vi "DL-SMART-MS-Modify-03-16.vi"() -> ()   [LabVIEW 2013]
uses:
  resources.vi
panel:
  out "status":string
  out "source":string
  out "DI":bool[](array[boolean])
  out "AI":dbl[](array[numeric])
  in  "message":string
  in  "offset Y":dbl format="%#_13g"
  in  "offset X":dbl format="%#_13g"
  out "ADC aquiring":bool
  out "motor moving":bool
  out "busy":bool
  out "Pul.HV-Real":dbl
  in  "ReportResult":bool
  out "Identify Spcetrum":cluster{"all rows":dbl[], "all rows":dbl[]}[](graph)=[{"all rows"=array[50131 elements], "all rows"=array[50131 elements]}, {"all rows"=array[360 elements], "all rows"=[0.0, -15.85746, 0.0, 0.0, -4.11823, 0.0, 0.0, -20.55303, 0.0, 0.0, -3.65583, 0.0, 0.0, -2.69345, 0.0, 0.0, -4.4706, 0.0, 0.0, -6.07537, 0.0, 0.0, -4.25015, 0.0, 0.0, -6.95758, 0.0, 0.0, -2.04252, 0.0, 0.0, -7.70754, 0.0, 0.0, -4.28864, 0.0, 0.0, -4.00869, 0.0, 0.0, -4.47517, 0.0, 0.0, -14.21368, 0.0, 0.0, -6.66072, 0.0, 0.0, -6.50078, 0.0, 0.0, -3.75903, 0.0, 0.0, -17.29715, 0.0, 0.0, -6.92254, 0.0, 0.0, -2.52353, 0.0, 0.0, -3.06405, 0.0, 0.0, -16.54211, 0.0, 0.0, -5.10076, 0.0, 0.0, -8.01669, 0.0, 0.0, -40.71695, 0.0, 0.0, -4.03763, 0.0, 0.0, -3.14159, 0.0, 0.0, -2.79298, 0.0, 0.0, -13.41979, 0.0, 0.0, -7.6464, 0.0, 0.0, -6.18956, 0.0, 0.0, -2.44901, 0.0, 0.0, -5.1704, 0.0, 0.0, -3.62455, 0.0, 0.0, -6.443, 0.0, 0.0, -24.18432, 0.0, 0.0, -37.78631, 0.0, 0.0, -4.28528, 0.0, 0.0, -3.21654, 0.0, 0.0, -3.13522, 0.0, 0.0, -4.8477, 0.0, 0.0, -3.80614, 0.0, 0.0, -8.10386, 0.0, 0.0, -2.86382, 0.0, 0.0, -17.8978, 0.0, 0.0, -4.74503, 0.0, 0.0, -9.4855, 0.0, 0.0, -5.75364, 0.0, 0.0, -80.29859, 0.0, 0.0, -5.18928, 0.0, 0.0, -28.13783, 0.0, 0.0, -6.84449, 0.0, 0.0, -4.07742, 0.0, 0.0, -2.99391, 0.0, 0.0, -4.60838, 0.0, 0.0, -3.257, 0.0, 0.0, -5.79015, 0.0, 0.0, -24.98325, 0.0, 0.0, -4.30828, 0.0, 0.0, -5.54625, 0.0, 0.0, -5.47663, 0.0, 0.0, -100.0001, 0.0, 0.0, -21.11295, 0.0, 0.0, -12.03347, 0.0, 0.0, -6.35092, 0.0, 0.0, -4.71483, 0.0, 0.0, -6.58836, 0.0, 0.0, -3.41548, 0.0, 0.0, -3.10072, 0.0, 0.0, -4.79955, 0.0, 0.0, -4.88109, 0.0, 0.0, -32.02295, 0.0, 0.0, -20.17071, 0.0, 0.0, -9.63953, 0.0, 0.0, -8.63946, 0.0, 0.0, -6.018, 0.0, 0.0, -6.3389, 0.0, 0.0, -14.67808, 0.0, 0.0, -6.22948, 0.0, 0.0, -4.9166, 0.0, 0.0, -44.64096, 0.0, 0.0, -5.6163, 0.0, 0.0, -8.56872, 0.0, 0.0, -11.1186, 0.0, 0.0, -4.42493, 0.0, 0.0, -15.45284, 0.0, 0.0, -2.99091, 0.0, 0.0, -18.05376, 0.0, 0.0, -3.06669, 0.0, 0.0, -35.88844, 0.0, 0.0, -19.12645, 0.0, 0.0, -3.20878, 0.0, 0.0, -2.61247, 0.0, 0.0, -7.79975, 0.0, 0.0, -5.8874, 0.0, 0.0, -5.7487, 0.0, 0.0, -5.43834, 0.0, 0.0, -21.69908, 0.0, 0.0, -64.96584, 0.0, 0.0, -5.77762, 0.0, 0.0, -5.55465, 0.0, 0.0, -4.62119, 0.0, 0.0, -3.61176, 0.0, 0.0, -6.99332, 0.0, 0.0, -4.34549, 0.0, 0.0, -15.09003, 0.0, 0.0, -6.25437, 0.0, 0.0, -21.85243, 0.0, 0.0, -13.24381, 0.0, 0.0, -3.94672, 0.0, 0.0, -3.90192, 0.0, 0.0, -11.14967, 0.0, 0.0, -83.69183, 0.0, 0.0, -11.19559, 0.0, 0.0, -7.83445, 0.0, 0.0, -3.14763, 0.0, 0.0, -6.44728, 0.0, 0.0, -5.69155, 0.0, 0.0, -4.00216, 0.0]}]
  in  "IdentifyMS":bool
  out "Spcetrum":cluster{"all rows":dbl[], "all rows":dbl[]}(graph)
  in  "Identification Record (鉴定记录表)":i32(listbox)=6
  in  "Identification Results (单靶鉴定结果)":i32(listbox)=2
  out "RedLaserEnergy":sgl=3.5 format="%.1f"
  in  "HVEnable":bool
  in  "CameraSet":bool
  out "执行进度栏":u8(slide) caption="Vaccum" scale=0.0..1.0
  out "GateClose":bool
  out "LaserOK":bool
  out "HV-OK":bool
  out "Vacuum-OK":bool
  in  "Tab Control":T1(tab)
  in  "SumShots (累加总数)":u32=300
  in  "Evalu. Shots (评估数)":u32=100
  in  "螺线半径步长":dbl=1.0
  in  "螺线旋转角度":u32=30
  in  "EditAutoTar":bool
  in  "SinglePoint":bool=TRUE
  in  "MultiPoints":bool
  in  "MultiTargets":bool
  in  "MCPHV-Set":dbl
  in  "LensHV-Set":dbl
  in  "Tar.HV-Set":dbl
  in  "Pul.HV-Set":dbl
  in  "PulseDelay":dbl
  in  "ADCFreq":dbl
  in  "MassRange":cluster{u64, u64}(slide) scale=0.0..100000.0
  in  "CH1_Coupling":u64(ring)=2 items=["Volt DC"=1, "Volt AC"=2, "Ampere DC"=4, "Ampere AC"=8, "Ohm"=16]
  in  "Channel 1_Range":dbl(ring)=4.0 items=["80 V"=80.0, "40 V"=40.0, "20 V"=20.0, "8 V"=8.0, "4 V"=4.0, "2 V"=2.0, "800 mV"=0.8, "400 mV"=0.4, "200 mV"=0.2]
  in  "Anal. Setting File":string="High Mass"
  in  "SettingFileSave":bool caption="TakeMS"
  in  "SettingFileAppl":bool caption="TakeMS"
  in  "SettingDel":bool caption="TakeMS"
  in  "RunADC":bool caption="TakeMS"
  in  "StopADC":bool caption="TakeMS"
  out "ADCstatus":bool
  out "TurboPower":dbl[unit]
  out "TurboVolts":dbl[unit]
  out "TurboCurr":dbl[unit]
  out "TurboAge":dbl[unit]
  out "TurboTemp":dbl[unit]
  in  "TurboRun":bool caption="TakeMS"
  in  "TurboStop":bool caption="TakeMS"
  out "TurboStatus":bool
  out "TurboSpeed":dbl(knob) scale=0.0..100.0
  in  "Vac_Prot.":bool
  in  "Turbo_Fore":bool
  in  "Main_Samp":bool
  in  "Samp_Atmos":bool
  in  "Fore_Samp":bool
  in  "激光运行":bool caption="TakeMS"
  out "发射":bool
  in  "频率/Hz":u8=60
  in  "激光衰减偏置当前":u8
  in  "激光衰减偏置 2":u8
  in  "激光衰减偏置":u8
  out "欠压":bool
  out "过热":bool
  out "待机":bool
  out "连接":bool
  out "LaserVolt":sgl format="%.1f"
  out "LaserTemp":sgl format="%.1f"
  out "Numeric":i64
  out "温警":bool
  out "开关损坏":bool
  out "开关监控":bool
  out "命令":bool
  in  "激光停止":bool caption="TakeMS"
  in  "GO":bool
  out "YH12下":dbl
  out "YA1上":dbl
  out "XH12右":dbl
  out "XA1左":dbl
  in  "Y+":bool
  in  "Y-":bool
  in  "X-":bool
  in  "X+":bool
  in  "Plat_To_Zero":bool caption="TakeMS"
  in  "Plat_Cal":bool caption="TakeMS"
  out "Ty":dbl
  out "Tx":dbl
  out "Y当前":dbl
  out "X当前":dbl
  out "移动":bool
  out "Y满":bool
  out "Y标":bool
  out "X标":bool
  out "Y0":bool
  out "X0":bool
  out "靶位In/Out":bool
  out "仓门":bool
  out "Y过热":bool
  out "X过热":bool
  out "通讯":bool
  in  "Operation Record":i32(listbox)
  in  "OptionRecordLoad 2":bool caption="TakeMS"
  in  "OptionRecordClear":bool caption="TakeMS"
  in  "CameraStart":bool
  in  "OpenCloseGate":bool
  out "Camera (摄像头)":dbl[][](graph)
  out "Tar.HV-Real":dbl
  out "LensHV-Real":dbl
  out "MCPHV-Real":dbl
  out "Lvaccum":dbl=0.83 format="%#_6e"
  out "Hvaccum":dbl=3.4e-05 format="%#_6e"
  in  "H12":bool
  in  "G12":bool
  in  "F12":bool
  in  "E12":bool
  in  "D12":bool
  in  "C12":bool
  in  "B12":bool
  in  "A12":bool
  in  "H11":bool
  in  "G11":bool
  in  "F11":bool
  in  "E11":bool
  in  "D11":bool
  in  "C11":bool
  in  "B11":bool
  in  "A11":bool
  in  "H10":bool
  in  "G10":bool
  in  "F10":bool
  in  "E10":bool
  in  "D10":bool
  in  "C10":bool
  in  "B10":bool
  in  "A10":bool
  in  "H9":bool
  in  "G9":bool
  in  "F9":bool
  in  "E9":bool
  in  "D9":bool
  in  "C9":bool
  in  "B9":bool
  in  "A9":bool
  in  "H8":bool
  in  "G8":bool
  in  "F8":bool
  in  "E8":bool
  in  "D8":bool
  in  "C8":bool
  in  "B8":bool
  in  "A8":bool
  in  "H7":bool
  in  "G7":bool
  in  "F7":bool
  in  "E7":bool
  in  "D7":bool
  in  "C7":bool
  in  "B7":bool
  in  "A7":bool
  in  "H6":bool
  in  "G6":bool
  in  "F6":bool
  in  "E6":bool
  in  "D6":bool
  in  "C6":bool
  in  "B6":bool
  in  "A6":bool
  in  "H5":bool
  in  "G5":bool
  in  "F5":bool
  in  "E5":bool
  in  "D5":bool
  in  "C5":bool
  in  "B5":bool
  in  "A5":bool
  in  "H4":bool
  in  "G4":bool
  in  "F4":bool
  in  "E4":bool
  in  "D4":bool
  in  "C4":bool
  in  "B4":bool
  in  "A4":bool
  in  "H3":bool
  in  "G3":bool
  in  "F3":bool
  in  "E3":bool
  in  "D3":bool
  in  "C3":bool
  in  "B3":bool
  in  "A3":bool
  in  "H2":bool
  in  "G2":bool
  in  "F2":bool
  in  "E2":bool
  in  "D2":bool
  in  "C2":bool
  in  "B2":bool
  in  "A2":bool
  in  "H1":bool
  in  "G1":bool
  in  "F1":bool
  in  "E1":bool
  in  "D1":bool
  in  "C1":bool
  in  "B1":bool
  in  "A1":bool
  out "Added":u32=300
  out "ith-Shot":dbl
  in  "Clear":bool caption="TakeMS"
  in  "Add":bool caption="TakeMS"
  in  "TakeMS-Stop":bool caption="TakeMS"
  in  "TakeMS-Run":bool caption="TakeMS"
  out "Sumshots":u32=300
  in  "SetLaserEnergy":dbl(slide) scale=0.0..10.0
  # "Laser (激光)"
  # "Camera (摄像头)"
  # "Mass Spectrum (质谱图)"
  # "Energy"
  # "mJ/pulse"
  # "Acq.(采谱)"
  # "1"
  # "2"
  # "3"
  # "4"
  # "5"
  # "6"
  # "7"
  # "8"
  # "9"
  # "10"
  # "11"
  # "12"
  # "Vacuum(真空)"
  # "A"
  # "Pa"
  # "High"
  # "B"
  # "Low"
  # "Pa"
  # "C"
  # "H.V.(高压)"
  # "D"
  # "Ident. (鉴定图)"
  # "MCP"
  # "V"
  # "E"
  # "Tar."
  # "V"
  # "F"
  # "Pul."
  # "V"
  # "G"
  # "Lens"
  # "V"
  # "H"
  # "Vauum (真空)"
  # "H.V. (高压)"
  # "Laser (激光)"
  # "Gate (仓门)"
  # "SinglePoint (单点)"
  # "MultiPoints (多点)"
  # "MultiTar. (多靶)"
  # "mm"
  # "度"
  # "H.V. (高压参数)"
  # "ADC(采集卡设置)"
  # "ADCFreq(采样)"
  # "MCP (探测器)"
  # "V"
  # "Hz"
  # "Tar. (靶)"
  # "V"
  # "Setting File(设置文件)"
  # "Coupling"
  # "Pulse (脉冲)"
  # "V"
  # "IntRange"
  # "V"
  # "Lens (透镜)"
  # "Delay (延时)"
  # "ns"
  # "Turbo Pump"
  # "Sole. Valves"
  # "自锁保护"
  # "机械/分子"
  # "℃"
  # "主仓/样仓"
  # "样仓/大气"
  # "机械/样仓"
  # "激光器状态"
  # "激光衰减器："
  # "发射次数："
  # "偏置："
  # "温度："
  # "摄氏度"
  # "范围："
  # "内部电源电压："
  # "V"
  # "当前："
  # "um"
  # "um"
  # "um"
  # "um"
  # "um"
  # "um"
  # "度"
  # "度"
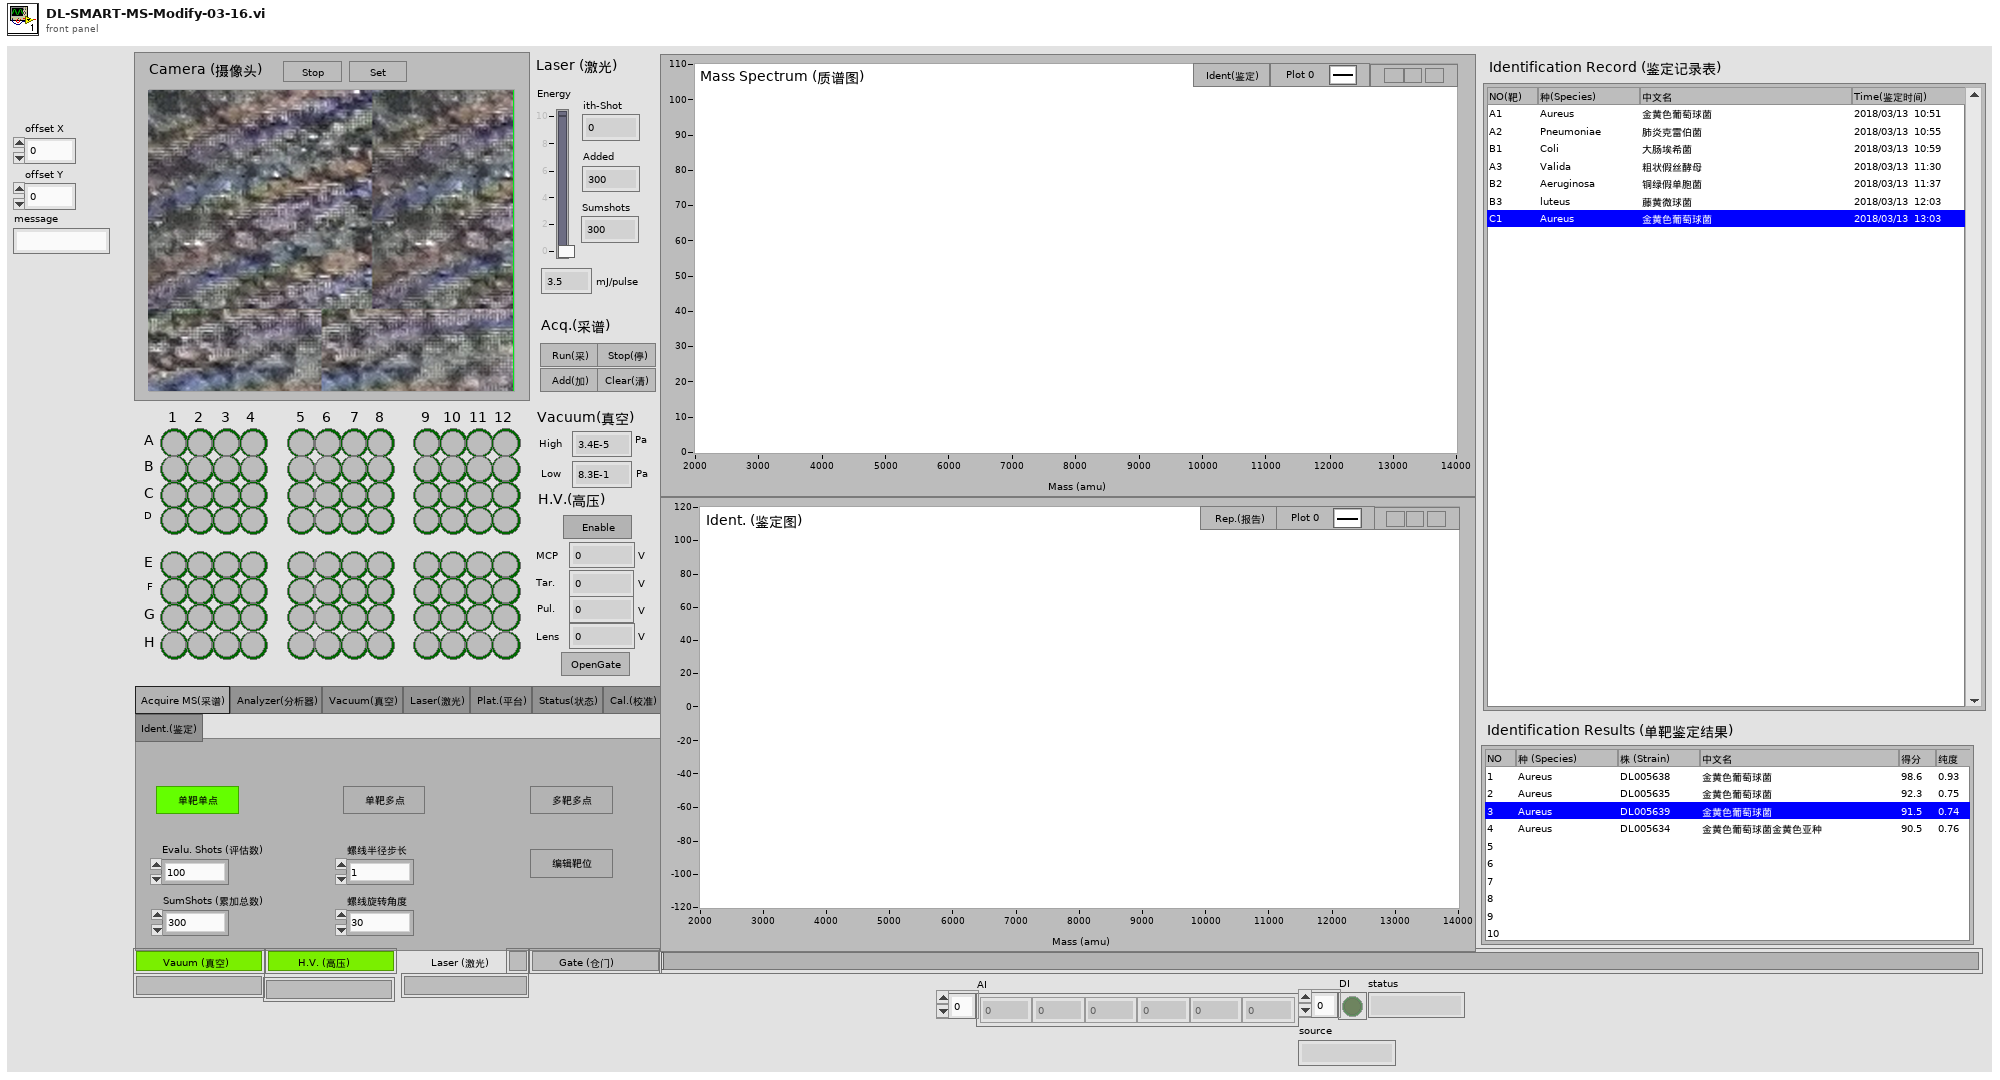
[diagram p1: front panel]
types:
  T1 = enum32{"Acquire MS(采谱)", "Analyzer(分析器)", "Vacuum(真空)", "Laser(激光)", "Plat.(平台)", "Status(状态)", "Cal.(校准)", "Ident.(鉴定)"}
  T2 = enum16{"adc aquire", "laser set", "motor move", "monitor", "wait", "stop"}
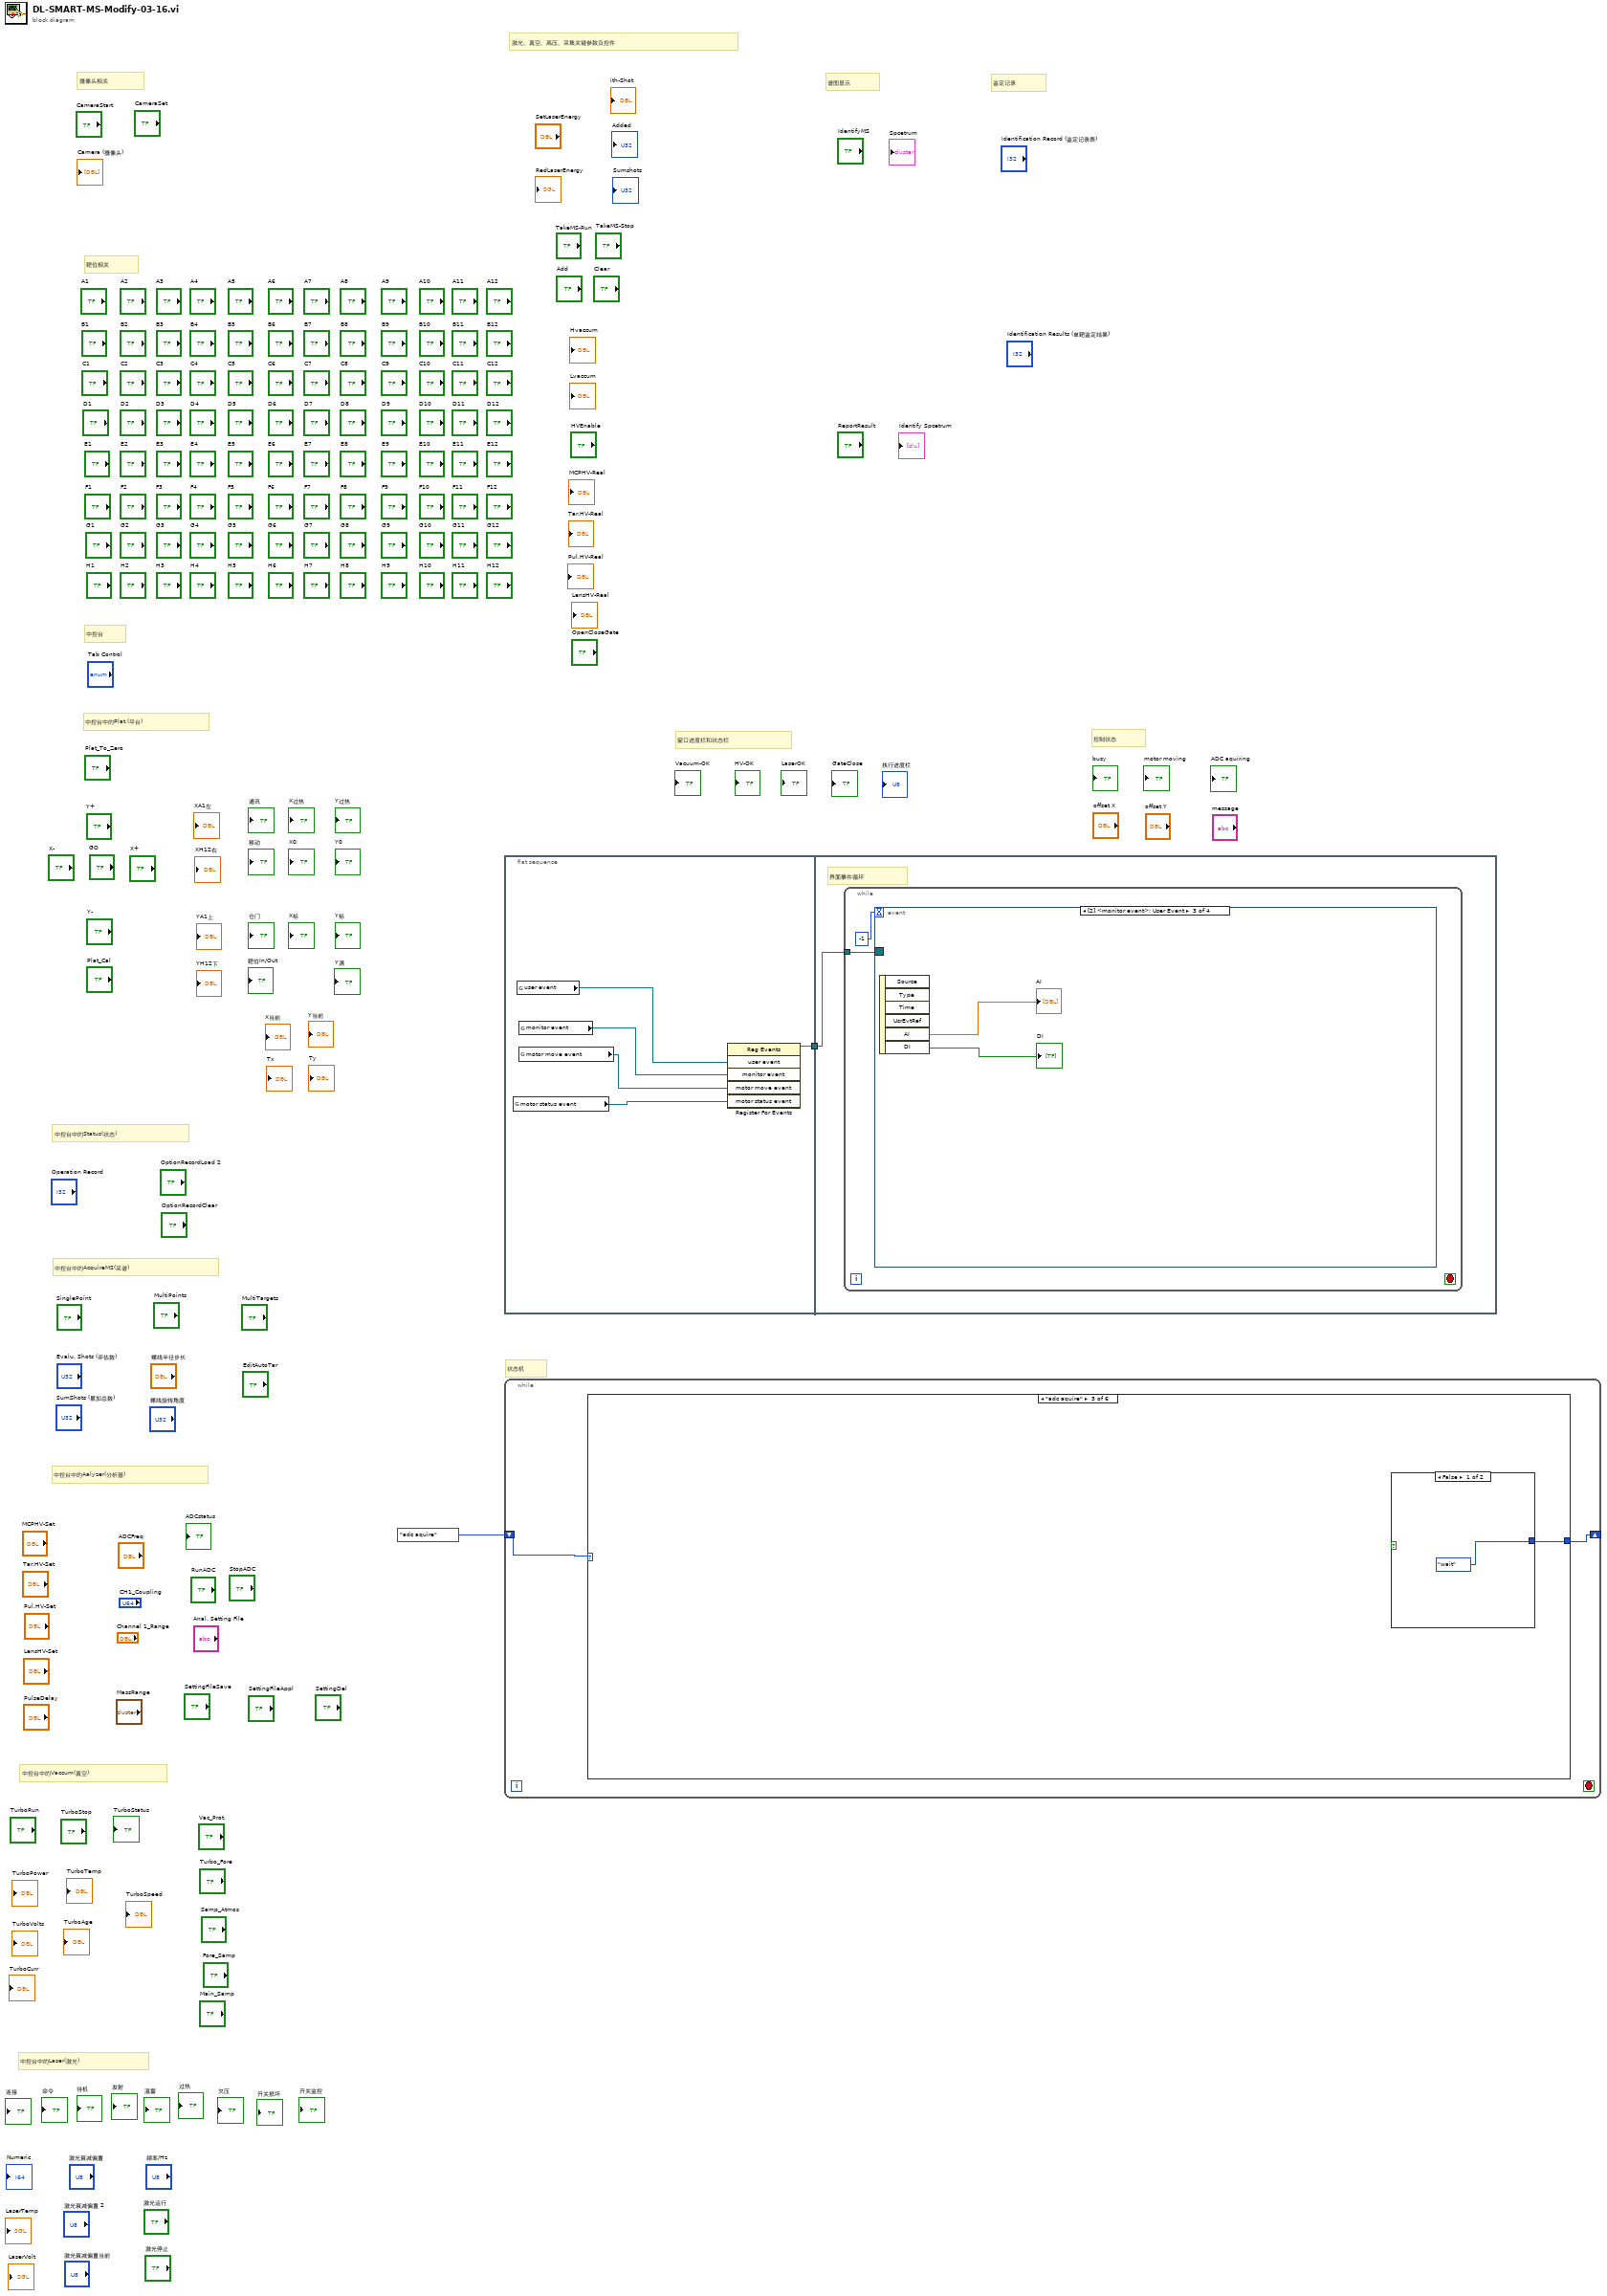
[diagram p0: block diagram]
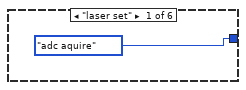
[diagram p2: hidden frame]
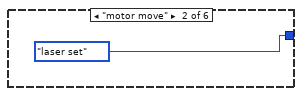
[diagram p3: hidden frame]
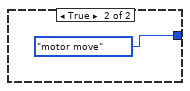
[diagram p4: hidden frame]
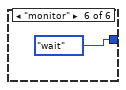
[diagram p7: hidden frame]
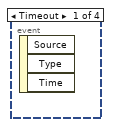
[diagram p8: hidden frame]
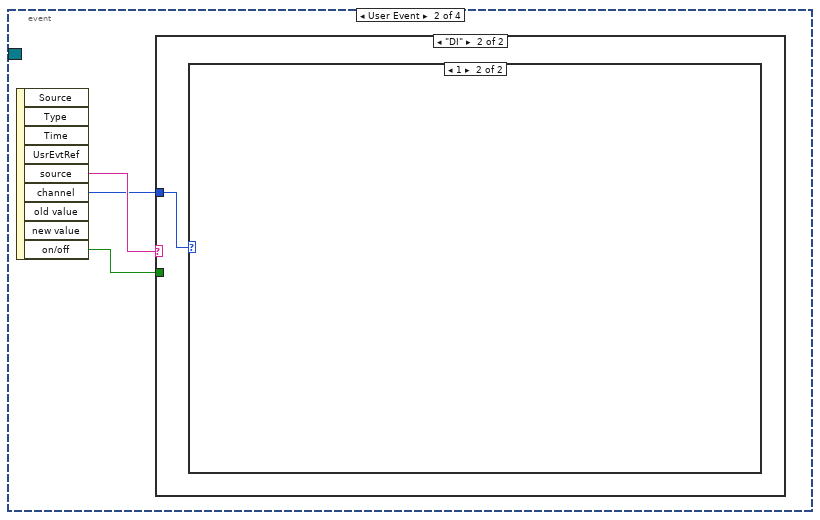
[diagram p9: hidden frame]
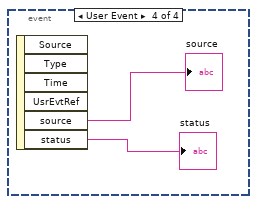
[diagram p12: hidden frame]
diagram:
  # "状态机"
  # "控制状态"
  # "鉴定记录"
  # "谱图显示"
  # "激光、真空、高压、采集关键参数及控件"
  # "窗口进度栏和状态栏"
  # "中控台中的Laser(激光)"
  # "中控台中的Vaccum(真空)"
  # "中控台中的Aalyzer(分析器)"
  # "中控台中的AcquireMS(采谱)"
  # "中控台中的Status(状态)"
  # "中控台中的Plat.(平台)"
  # "中控台"
  # "靶位相关"
  # "摄像头相关"
  n1 = flat-sequence {
    tunnel: [w7] -> w2
    tunnel: w2 -> [w8]
    frame #0 {
      n2 = global read "resources.vi" "motor status event"() -> (w3:refnum<user-event>)
      n3 = global read "resources.vi" "user event"() -> (w6:refnum<user-event>)
      n4 = global read "resources.vi" "monitor event"() -> (w5:refnum<user-event>)
      n5 = global read "resources.vi" "motor move event"() -> (w4:refnum<user-event>)
      n6 = register-events(w6, w5, w4, w3) -> (reference out=w7:refnum<event-registration>)  [unwired: 2 in, 1 out]
    }
    frame #1 {
      # "界面事件循环"
      n7 = while {
        tunnel: w8 -> [w10]
        stop <- _ stop-if-true
        n8 = event shown="[2] <monitor event>: User Event" {
          selector: w10 -> [_ _ _ _]
          dyn-events: _ -> [_ _ _ _]
          timeout: -1 -> [_ _ _ _]
          event Timeout {
            n9 = event-data() -> ()  [unwired: 1 in, 3 out]
          }
          event User Event {
            n10 = event-data() -> ("source"=w13:string, "channel"=w12:i32, "on/off"=w11:bool)  [unwired: 1 in, 6 out]
            n11 = case shown="\"DI\"" w13 {
              tunnel: w12 -> [_ w14]
              tunnel: w11 -> [_ _]
              frame "AI" {
              }
              frame "DI" {
                n12 = case shown="1" w14 {
                  frame 0, Default {
                  }
                  frame 1 {
                  }
                }
              }
            }
          }
          event User Event {
            n13 = event-data() -> ("AI"=→"AI":dbl[], "DI"=→"DI":bool[])  [unwired: 1 in, 4 out]
          }
          event User Event {
            n14 = event-data() -> ("source"=→"source":string, "status"=→"status":string)  [unwired: 1 in, 4 out]
          }
        }
      }
    }
  }
  n15 = while {
    shift-right: [w19] -> _
    shift-left: T2."adc aquire" ("状态") -> [w20]
    stop <- _ stop-if-true
    n16 = case shown="\"adc aquire\"" w20 {
      tunnel: [T2."adc aquire" ("状态") T2."laser set" ("状态") w23 _ _ T2."wait" ("状态")] -> w19
      frame "laser set" {
      }
      frame "motor move" {
      }
      frame "adc aquire" {
        n17 = case shown="False" {
          selector: _ -> [_ _]
          tunnel: [T2."wait" ("状态") T2."motor move" ("状态")] -> w23
          frame False {
          }
          frame True {
          }
        }
      }
      frame "wait" {
      }
      frame "stop" {
      }
      frame "monitor" {
      }
    }
  }
